vi "Read Talons.vi"   [LabVIEW 2018]
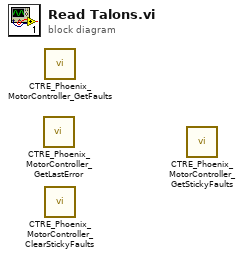
[diagram p0: block diagram]
diagram:
  n1 = call <vilib>:"CTRE_Phoenix_MotorController_GetLastError.vi"() -> ()  [unwired: 13 in, 3 out]
  n2 = call <vilib>:"CTRE_Phoenix_MotorController_GetFaults.vi"() -> ()  [unwired: 9 in, 3 out]
  n3 = call <vilib>:"CTRE_Phoenix_MotorController_ClearStickyFaults.vi"() -> ()  [unwired: 10 in, 2 out]
  n4 = call <vilib>:"CTRE_Phoenix_MotorController_GetStickyFaults.vi"() -> ()  [unwired: 9 in, 3 out]
